vi "escapi_close_camera.vi"(8 "error in (no error)":errorcluster, 11 "camera_name":string) -> (0 "error out":errorcluster)   [LabVIEW 2022 SP3, in "Vision.lvlib"]
uses:
  Vision.lvlib
  bin/Vision.dll
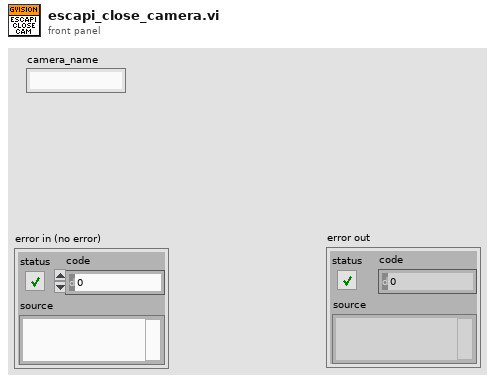
[diagram p1: front panel]
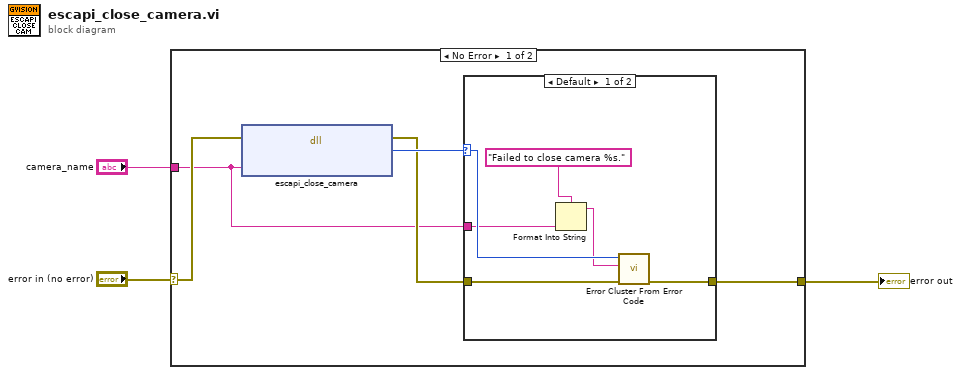
[diagram p0: block diagram]
diagram:
  n1 = case shown="No Error" "error in (no error)" {
    selector: "error in (no error)" -> [w8 w16]
    tunnel: [w5 w16] -> w1
    tunnel: "camera_name" -> [w4 _]
    frame No Error {
      n2 = dll-call lib="C:/Users/Caleb/Desktop/nebraska-silicon-lab/pixel-gantry-extra/LV/bin/Vision.dll" fn="escapi_close_camera"(error in=w8, "camera_name"=w4) -> (error out=w6:errorcluster, "return type"=w7:i32)  [unwired: 3 in, 1 out]
      n3 = case shown="Default" w7 {
        selector: w7 -> [w12 _]
        tunnel: w6 -> [w14 w15]
        tunnel: [w13 w15] -> w5
        tunnel: w4 -> [w10 _]
        frame Default {
          n4 = Format Into String(format string="Failed to close camera %s." ("error message (\"\")"), w10) -> (resulting string=w9:string)  [unwired: 2 in, 1 out]
          n5 = call <vilib>:"Error Cluster From Error Code.vi"("error in (no error)"=w14, "error message (\"\")"=w9, "error code (0)"=w12) -> ("error out"=w13:errorcluster)  [unwired: 6 in]
        }
        frame 0 {
        }
      }
    }
    frame Error {
    }
  }
  "error out" <- w1
